vi "NI_PCIE_4353_32TC.vi"(11 "Queue Ref In":T1={"UI"=refnum, "Message"=refnum, "Data"=refnum, "Caller"=refnum, "Name"="000 Common", "Data Path"=path "", "Class Path"=path "", "SubPanel"=refnum, "Project Name"="", "MNT"="", "Title"="", "Data Source"=refnum, "Queue List"={}, "VI"=refnum, "UE"=refnum}) -> ()   [LabVIEW 2020]
doc: "PCIE_6509"
uses:
  Alin/QMH/000 Module Data Type.ctl
  Alin/QMH/Queue Message.ctl
  9999 SubVI/Global/Data Global/SDQ Data Type.ctl
  <vilib>/DAQmx/read.llb/DAQmx Read (Analog 1D DBL NChan 1Samp).vi
  <vilib>/DAQmx/create/channels.llb/DAQmx Create Channel (AI-Temperature-Thermocouple).vi
  <vilib>/DAQmx/miscellaneous.llb/DAQmx Fill In Error Info.vi
  <resource>/objmgr/daqmx.rc
panel:
  out "Type":map{string, string}(c390)
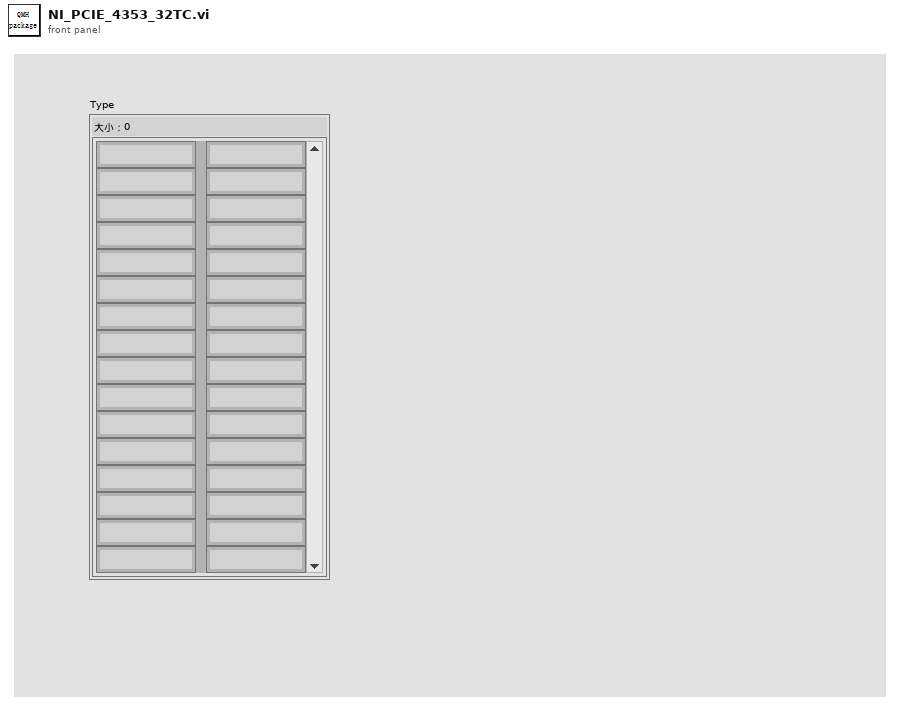
[diagram p1: front panel]
types:
  T1 = typedef "000 Module Data Type.ctl" = cluster{"UI":refnum<queue>, "Message":refnum<queue>, "Data":refnum<queue>, "Caller":refnum<queue>, "Name":string, "Data Path":path, "Class Path":path, "SubPanel":refnum<vi>, "Project Name":string, "MNT":string, "Title":string, "Data Source":refnum<queue>, "Queue List":map{string, refnum<queue>}, "VI":refnum<vi>, "UE":refnum<user-event>}
  T2 = typedef "SDQ Data Type.ctl" = cluster{"CAN Length":string, "CAN Name":string, "CAN ID":string, "CAN Type":string, "Test Item":string, "Byte Order":string, "Instruction":string, "Control Type":string, "Group":string, "Offset":dbl, "Coefficient":dbl, "Write Enable":bool, "Lable Type":string, "Key?":string, "Set Value":string, "Upper":dbl, "Lower":dbl, "Unit":string, "Formula":string, "Test Item Type":string, "Length":i32, "Address":string, "Name":string, "Identifier":string, "Data Type":string, "Enumerate?":string, "Enumerate List":string, "Data":string, "Source":string}
  T3 = cluster{"Queue":T1, "Delay":cluster{"Count Time(ms)":u32, "Delay Time(ms)":u32, "Next":string}, "Data":map{string, T2}, "PCIE_6509":cluster{"Port":string, "Task":refnum<k21>}, "IDS":string[], "Type":map{string, string}}
  T4 = typedef "005 Data Source Type.ctl" = cluster{"Device Name":string, "Device Model":string, "Device Driver":string, "IP Address":string, "Port":string, "Remark":string, "Enable":string, "Path":string}
  T5 = cluster{"Name":string, "Type":map{string, string}}
  T6 = typedef "eventvkey.ctl" = enum16{"ASCII", "Enter", "Return", "Shift", "Ctrl", "Alt", "Cmd", "Opt", "Caps", "NumLock", "Clear", "Break", "Up", "Down", "Left", "Right", "Insert", "Delete", "Home", "End", "PageUp", "PageDown", "Escape", "Help", "Pause", "ScrollLock", "F1", "F2", "F3", "F4", "F5", "F6", "F7", "F8", "F9", "F10", "F11", "F12", "F13", "F14", "F15", "F16", "F17", "F18", "F19", "F20", "F21", "F22", "F23", "F24", "Play", "VolumeUp", "VolumeDown", "Mute", "Two Byte Char"}
  T7 = cluster{"Shift":bool, "Ctrl":bool, "Alt":bool, "Cmd":bool, "Opt":bool}
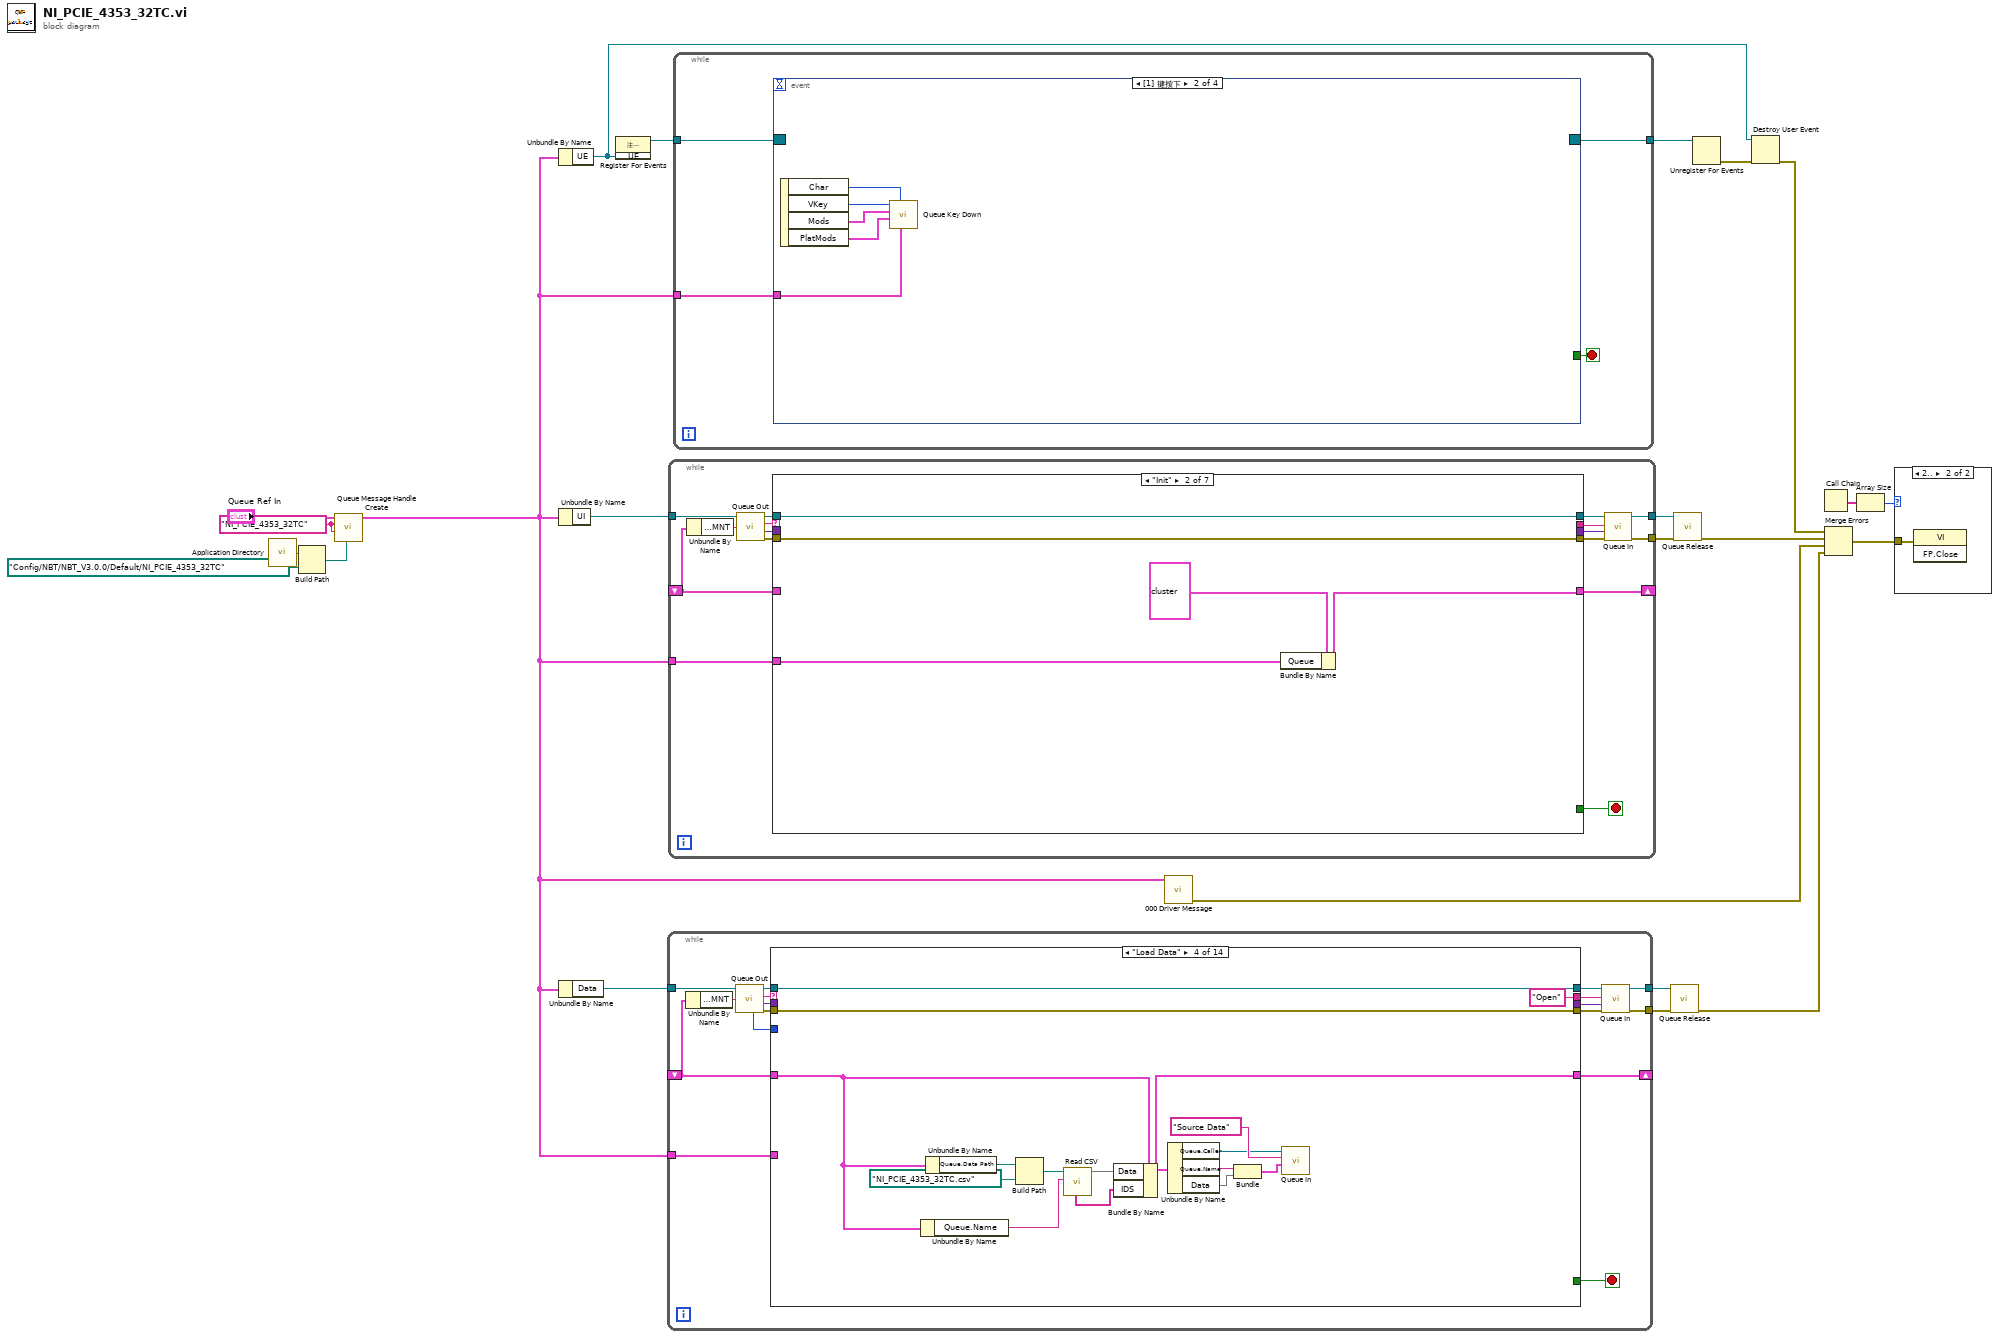
[diagram p0: block diagram]
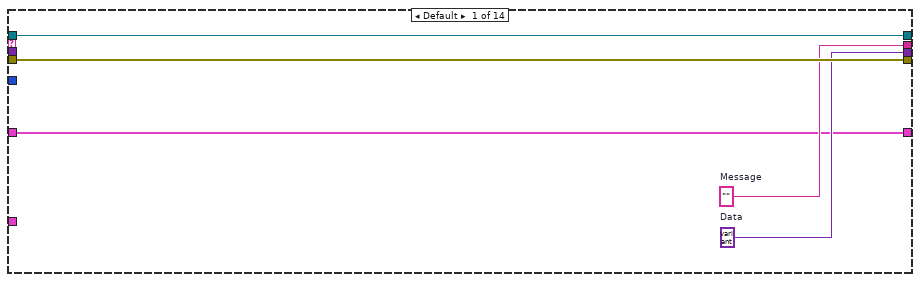
[diagram p2: hidden frame]
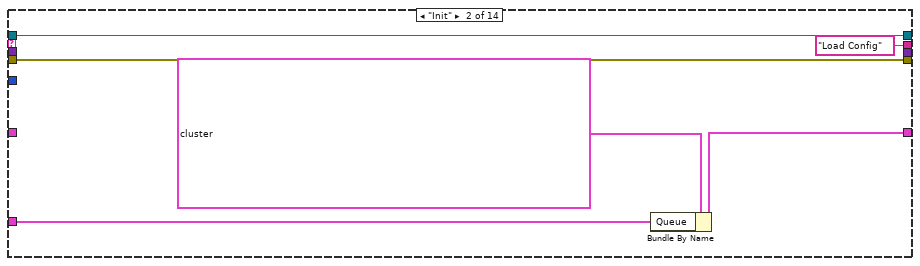
[diagram p3: hidden frame]
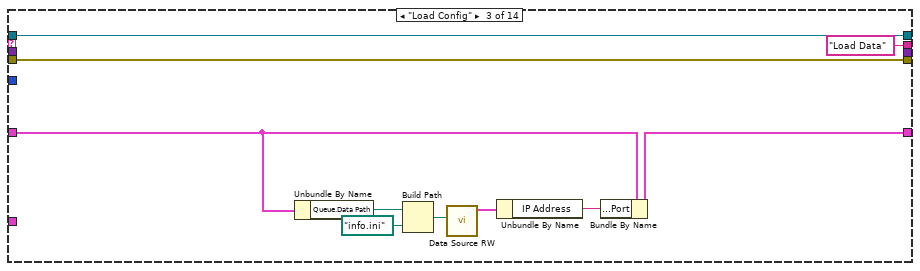
[diagram p4: hidden frame]
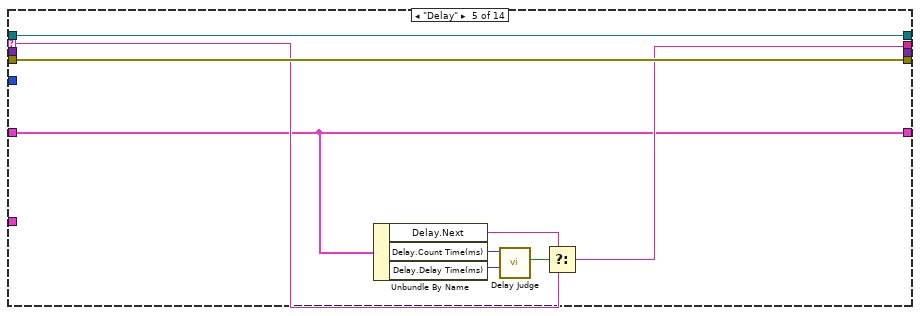
[diagram p5: hidden frame]
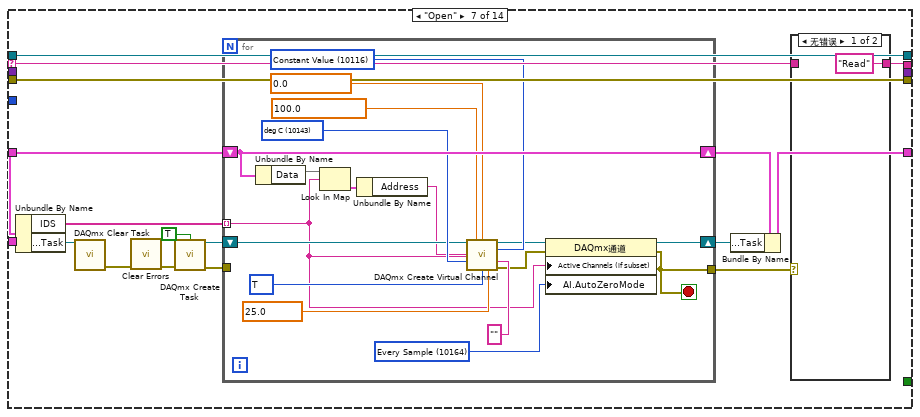
[diagram p7: hidden frame]
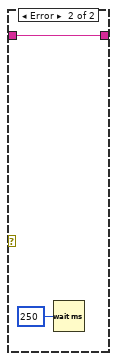
[diagram p8: hidden frame]
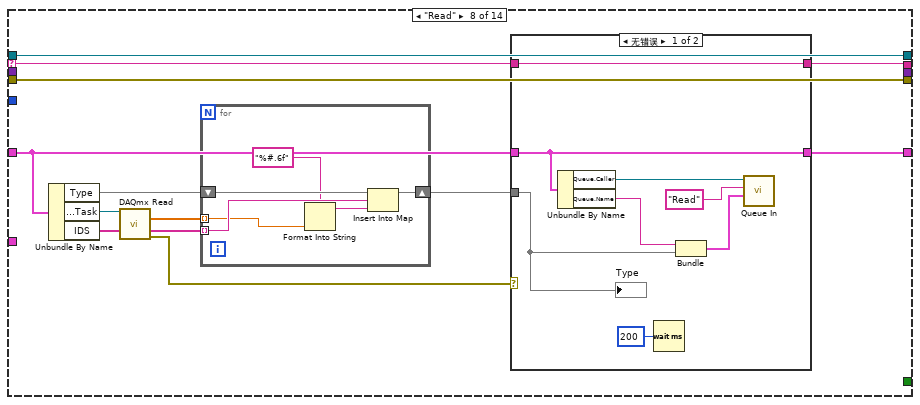
[diagram p9: hidden frame]
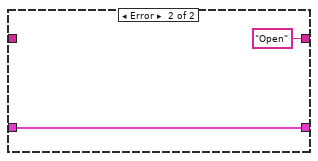
[diagram p10: hidden frame]
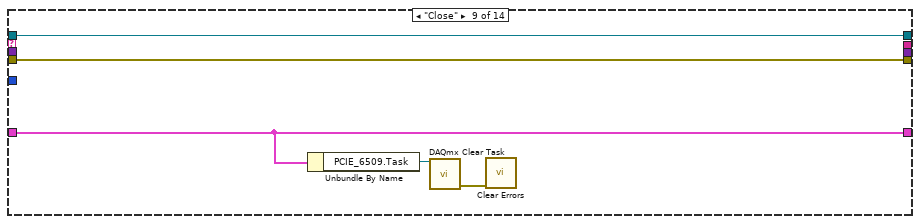
[diagram p11: hidden frame]
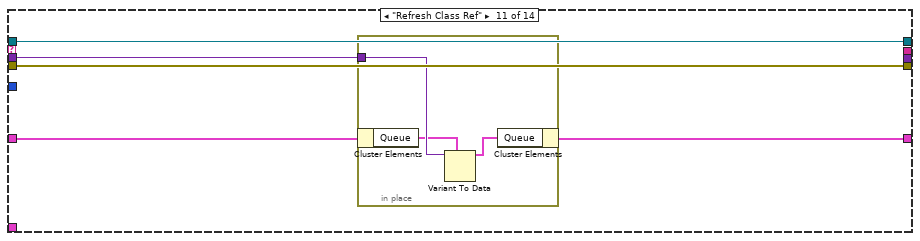
[diagram p13: hidden frame]
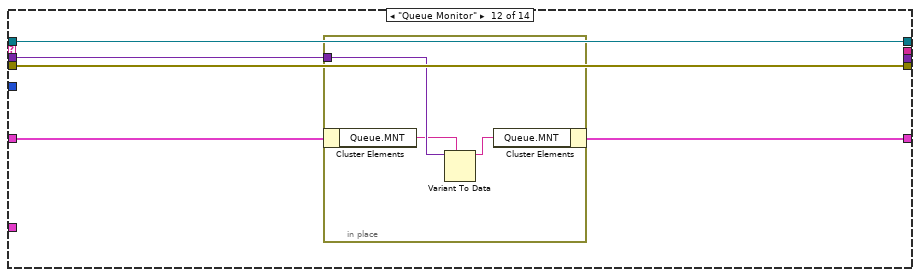
[diagram p14: hidden frame]
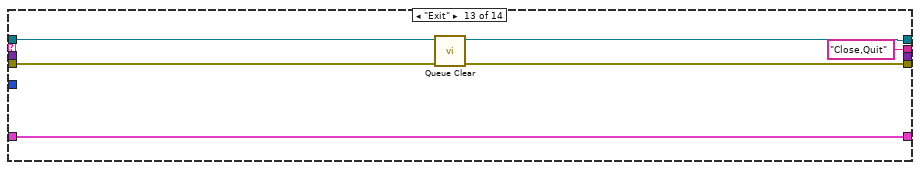
[diagram p15: hidden frame]
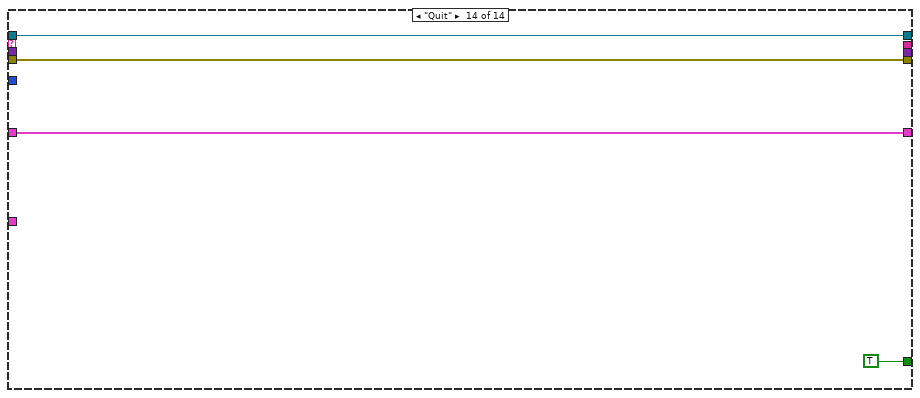
[diagram p16: hidden frame]
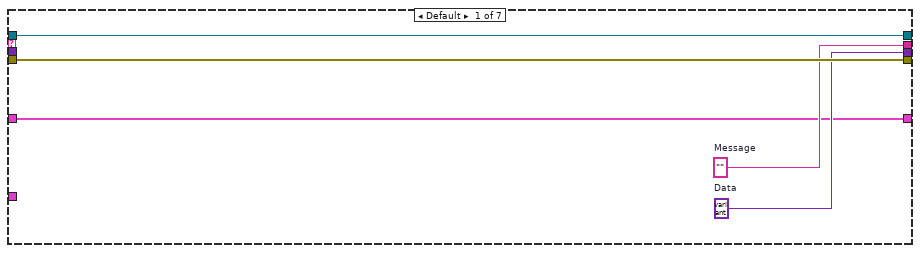
[diagram p18: hidden frame]
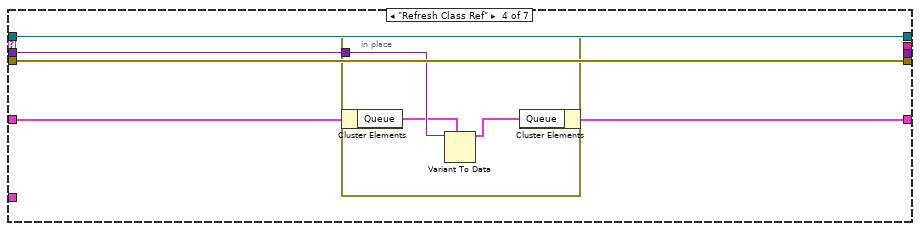
[diagram p20: hidden frame]
diagram:
  w1 = "NI_PCIE_4353_32TC" ("Title")
  n1 = call <vilib>:"Application Directory.vi"() -> ("Application Directory"=w4:path)
  n2 = Build Path(base path=w4, name or relative path=path "Config/NBT/NBT_V3.0.0/Default/NI_PCIE_4353_32TC" ("名称或相对路径")) -> (appended path=w2:path)
  n3 = call "Queue Message Handle Create.vi"("Data Path"=w2, "Name"=w1, "Title"=w1, "Queue Ref In"="Queue Ref In") -> ("Queue Ref Out"=w5:T1)  [unwired: 6 in, 1 out]
  n4 = Unbundle By Name(w5) -> ("UE"=w7:refnum<user-event>)
  n5 = Unbundle By Name(w5) -> ("UI"=w18:refnum<queue>)
  n6 = Unbundle By Name(w5) -> ("Data"=w10:refnum<queue>)
  n7 = register-events(w7) -> (reference out=w23:refnum<event-registration>)  [unwired: 2 in, 1 out]
  n8 = while {
    tunnel: w10 -> [w36]
    tunnel: [w33] -> w12
    tunnel: [w32] -> w11
    shift-right: [w28] -> _
    shift-left: _ -> [w25]
    tunnel: w5 -> [w24]
    stop <- w40 stop-if-true
    n9 = Unbundle By Name(w25) -> ("Queue.MNT"=w26:string)
    n10 = call "Queue Out.vi"("Monitor"=w26, "Queue In"=w36) -> ("error out"=w39:errorcluster, "Data"=w37:variant, "Message"=w38:string, "Queue Out"=w35:refnum<queue>, "Queue NUmber"=w27:i32)  [unwired: 5 in]
    n11 = case shown="\"Load Data\"" w38 {
      selector: w38 -> [_ _ _ _ w79 _ w95 w131 _ _ _ _ _ _]
      tunnel: w35 -> [w45 w51 w61 w77 w86 w89 w105 w138 w159 w162 w167 w175 w183 w187]
      tunnel: w39 -> [w44 w50 w60 w76 w85 w88 w104 w137 w158 w161 w166 w174 w181 w188]
      tunnel: [w45 w51 w61 w77 w86 w89 w105 w138 w159 w162 w167 w175 w182 w187] -> w34
      tunnel: [w44 w50 w60 w76 w85 w88 w104 w137 w158 w161 w166 w174 w180 w188] -> w31
      tunnel: [w43 "Load Config" ("Next") "Load Data" ("Next") "Open" ("Next") w80 _ w94 w130 _ _ _ _ "Close,Quit" _] -> w30
      tunnel: [_ _ _ _ _ _ _ _ _ _ _ _ _ TRUE] -> w40
      tunnel: [w42 _ _ _ _ _ _ _ _ _ _ _ _ _] -> w29
      tunnel: w37 -> [_ _ _ _ _ _ _ _ _ _ w163 w171 _ _]
      tunnel: [w41 w47 w53 w66 w78 w87 w102 w132 w157 w160 w164 w172 w179 w185] -> w28
      tunnel: w25 -> [w41 _ w58 w63 w78 w87 w92 w133 w157 w160 w165 w173 w179 w185]
      tunnel: w27 -> [_ _ _ _ _ _ _ _ _ _ _ _ _ _]
      tunnel: w24 -> [_ w46 _ _ _ _ _ _ _ _ _ _ _ _]
      frame Default {
        w42 = variant  # Data
        w43 = ""  # Message
      }
      frame "Init" {
        n12 = Bundle By Name(cluster=T3 {"Queue"={"UI"=refnum, "Message"=refnum, "Data"=refnum, "Caller"=refnum, "Name"="000 Common", "Data Path"=path "", "Class Path"=path "", "SubPanel"=refnum, "Project Name"="", "MNT"="", "Title"="", "Data Source"=refnum, "Queue List"={}, "VI"=refnum, "UE"=refnum}, "Delay"={"Count Time(ms)"=250, "Delay Time(ms)"=250, "Next"="Receive Data,Delay"}, "Data"={}, "PCIE_6509"={"Port"="", "Task"=""}, "IDS"=[], "Type"={}}, "Queue"=w46) -> (w47:T3)
      }
      frame "Load Config" {
        n13 = Unbundle By Name(w58) -> ("Queue.Data Path"=w57:path)
        n14 = Build Path(base path=w57, name or relative path=path "info.ini" ("名称或相对路径")) -> (appended path=w55:path)
        n15 = call "Data Source RW.vi"("Source Path"=w55) -> ("Data Type Out"=w54:T4)  [unwired: 7 in, 3 out]
        n16 = Unbundle By Name(w54) -> ("IP Address"=w52:string)
        n17 = Bundle By Name(cluster=w58, "PCIE_6509.Port"=w52) -> (w53:T3)
      }
      frame "Load Data" {
        n18 = Unbundle By Name(w63) -> ("Queue.Name"=w62:string)
        n19 = Unbundle By Name(w63) -> ("Queue.Data Path"=w75:path)
        n20 = Build Path(base path=w75, name or relative path=path "NI_PCIE_4353_32TC.csv" ("名称或相对路径")) -> (appended path=w73:path)
        n21 = call "Read CSV.vi"("Source"=w62, "Data Path"=w73) -> (3:"Identifiers Out"=w72:map{string, T2}, 6:"Identifiers Out"=w65:string[])  [unwired: 2 in, 6 out]
        n22 = Bundle By Name(cluster=w63, "Data"=w72, "IDS"=w65) -> (w66:T3)
        n23 = Unbundle By Name(w66) -> ("Queue.Caller"=w67:refnum<queue>, "Queue.Name"=w71:string, "Data"=w69:map{string, T2})
        n24 = Bundle("Name"=w71, "Data"=w69) -> (w70:cluster{"Name":string, "Data":map{string, T2}})  [unwired: 1 in]
        n25 = call "Queue In.vi"("Data"=w70, "Message"="Source Data", "Queue In"=w67) -> ()  [unwired: 7 in, 2 out]
      }
      frame "Delay" {
        n26 = Unbundle By Name(w78) -> ("Delay.Next"=w84:string, "Delay.Count Time(ms)"=w81:u32, "Delay.Delay Time(ms)"=w82:u32)
        n27 = call "Delay Judge.vi"("Delay Time(ms)"=w82, "Count Time(ms)"=w81) -> ("Time Out?"=w83:bool)  [unwired: 5 in, 4 out]
        n28 = Select(t=w84, s=w83, f=w79) -> (s? t:f=w80:string)
      }
      frame "===Driver====" {
      }
      frame "Open" {
        n29 = Unbundle By Name(w92) -> ("IDS"=w93:string[], "PCIE_6509.Task"=w101:refnum<k21>)
        n30 = call <vilib>:"DAQmx Clear Task.vi"("task in"=w101) -> ("error out"=w100:errorcluster)  [unwired: 14 in]
        n31 = call <vilib>:"Clear Errors.vi"("error in (no error)"=w100) -> ("error out"=w99:errorcluster)  [unwired: 5 in, 1 out]
        n32 = call <vilib>:"DAQmx Create Task.vi"("auto cleanup"=TRUE, "error in"=w99) -> ("task out"=w98:refnum<k21>, "error out"=w90:errorcluster)  [unwired: 12 in]
        n33 = for {
          shift-right: [w113] -> w97
          shift-left: w98 -> [w116]
          tunnel: [w111] -> w96
          tunnel: w93 -> [w110] mode=indexing
          shift-right: [w126] -> w91
          shift-left: w92 -> [w126]
          tunnel: w90 -> [_]
          stop <- w111 stop-if-true
          w109 = 10164 items=["None"=10230, "Once"=10244, "Every Sample"=10164] ("AutoZeroMode")
          w120 = 10143 items=["deg C"=10143, "deg F"=10144, "Kelvins"=10325, "deg R"=10145, "From Custom Scale"=10065] ("units")
          w118 = 10086 items=["J"=10072, "K"=10073, "N"=10077, "R"=10082, "S"=10085, "T"=10086, "B"=10047, "E"=10055] ("thermocouple type")
          w121 = u32 10116 items=["Internal"=10200, "Constant Value"=10116, "Channel"=10113] ("cjc source")
          n34 = Unbundle By Name(w126) -> ("Data"=w125:map{string, T2})
          n35 = Look In Map(map=w125, key=w110) -> (value=w124:T2)  [unwired: 1 in, 1 out]
          n36 = Unbundle By Name(w124) -> ("Address"=w115:string)
          n37 = call-poly <vilib>:"DAQmx Create Virtual Channel.vi"("task in"=w116, "maximum value"=100.0, "minimum value"=0.0, "physical channels"=w115, "cjc source"=w121, "name to assign"=w110, "units"=w120, "cjc channel"="", "thermocouple type"=w118, "cjc value"=25.0) -> ("task out"=w114:refnum<k21>, "error out"=w112:errorcluster)  [unwired: 4 in]
          n38 = property class="DAQmx通道"(reference=w114, error in=w112, "Active Channels (if subset)"=w110, "AI.AutoZeroMode"=w109) -> (reference out=w113:refnum<k21>, error out=w111:errorcluster)
        }
        n39 = Bundle By Name(cluster=w91, "PCIE_6509.Task"=w97) -> (w102:T3)
        n40 = case shown="无错误" w96 {
          tunnel: w95 -> [_ w108]
          tunnel: ["Read" w108] -> w94
          frame No Error {
          }
          frame Error {
            n41 = Wait (ms)(milliseconds to wait=u32 250 ("等待时间（毫秒）")) -> ()  [unwired: 1 out]
          }
        }
      }
      frame "Read" {
        n42 = Unbundle By Name(w133) -> ("Type"=w135:map{string, string}, "PCIE_6509.Task"=w129:refnum<k21>, "IDS"=w136:string[])
        n43 = call-poly <vilib>:"DAQmx Read.vi"("task/channels in"=w129) -> ("data"=w127:dbl[], "error out"=w128:errorcluster)  [unwired: 12 in, 1 out]
        n44 = for {
          tunnel: w136 -> [w153] mode=indexing
          shift-right: [w152] -> w134
          shift-left: w135 -> [w154]
          tunnel: w127 -> [w150] mode=indexing
          n45 = Format Into String(format string="%#.6f" ("格式字符串"), w150) -> (resulting string=w149:string)  [unwired: 2 in, 1 out]
          n46 = Insert Into Map(map in=w154, key=w153, value=w149) -> (map out=w152:map{string, string})  [unwired: 2 out]
        }
        n47 = case shown="无错误" w128 {
          tunnel: w134 -> [w139 _]
          tunnel: w133 -> [w146 w148]
          tunnel: [w146 w148] -> w132
          tunnel: w131 -> [w141 _]
          tunnel: [w141 "Open"] -> w130
          frame No Error {
            n48 = Unbundle By Name(w146) -> ("Queue.Caller"=w145:refnum<queue>, "Queue.Name"=w143:string)
            n49 = Wait (ms)(milliseconds to wait=u32 200 ("等待时间（毫秒）")) -> ()  [unwired: 1 out]
            n50 = Bundle("Name"=w143, "Type"=w139) -> (w142:T5)  [unwired: 1 in]
            n51 = call "Queue In.vi"("Data"=w142, "Message"="Read", "Queue In"=w145) -> ()  [unwired: 7 in, 2 out]
            "Type" <- w139
          }
          frame Error {
          }
        }
      }
      frame "Close" {
        n52 = Unbundle By Name(w157) -> ("PCIE_6509.Task"=w156:refnum<k21>)
        n53 = call <vilib>:"DAQmx Clear Task.vi"("task in"=w156) -> ("error out"=w155:errorcluster)  [unwired: 14 in]
        n54 = call <vilib>:"Clear Errors.vi"("error in (no error)"=w155) -> ()  [unwired: 5 in, 2 out]
      }
      frame "====System====" {
      }
      frame "Refresh Class Ref" {
        n55 = in-place {
          in-place-border: w163 -> [w170]
          n56 = in-place-cluster #1(w165) -> ("Queue"=w169:T1)
          n57 = Variant To Data(type=w169, Variant=w170) -> (data=w168:T1)  [unwired: 1 in, 1 out]
          n58 = in-place-cluster #1("Queue"=w168) -> (w164:T3)
        }
      }
      frame "Queue Monitor" {
        n59 = in-place {
          in-place-border: w171 -> [w178]
          n60 = in-place-cluster #2(w173) -> ("Queue.MNT"=w177:string)
          n61 = Variant To Data(type=w177, Variant=w178) -> (data=w176:string)  [unwired: 1 in, 1 out]
          n62 = in-place-cluster #2("Queue.MNT"=w176) -> (w172:T3)
        }
      }
      frame "Exit" {
        n63 = call "Queue Clear.vi"("error in (no error)"=w181, "Queue In"=w183) -> ("error out"=w180:errorcluster, "Queue Out"=w182:refnum<queue>)  [unwired: 8 in]
      }
      frame "Quit" {
      }
    }
    n64 = call "Queue In.vi"("error in (no error)"=w31, "Data"=w29, "Message"=w30, "Queue In"=w34) -> ("error out"=w32:errorcluster, "Queue Out"=w33:refnum<queue>)  [unwired: 6 in]
  }
  n65 = while {
    tunnel: w18 -> [w200]
    tunnel: [w197] -> w20
    tunnel: [w196] -> w19
    shift-right: [w192] -> _
    shift-left: _ -> [w191]
    tunnel: w5 -> [w189]
    stop <- w204 stop-if-true
    n66 = Unbundle By Name(w191) -> ("Queue.MNT"=w190:string)
    n67 = call "Queue Out.vi"("Monitor"=w190, "Queue In"=w200) -> ("error out"=w203:errorcluster, "Data"=w201:variant, "Message"=w202:string, "Queue Out"=w199:refnum<queue>)  [unwired: 5 in, 1 out]
    n68 = case shown="\"Init\"" w202 {
      selector: w202 -> [_ _ _ _ _ w236 _]
      tunnel: w199 -> [w209 w214 w217 w222 w230 w243 w249]
      tunnel: w203 -> [w208 w213 w216 w221 w229 w241 w250]
      tunnel: [w209 w214 w217 w222 w230 w242 w249] -> w198
      tunnel: [w208 w213 w216 w221 w229 w240 w250] -> w195
      tunnel: [w207 _ _ _ _ "Quit" _] -> w194
      tunnel: [_ _ _ _ _ _ TRUE] -> w204
      tunnel: [w206 _ _ _ _ _ _] -> w193
      tunnel: w201 -> [_ _ _ w218 w226 _ _]
      tunnel: [w205 w211 w215 w219 w227 w235 w247] -> w192
      tunnel: w191 -> [w205 _ w215 w220 w228 w235 w247]
      tunnel: w189 -> [_ w210 _ _ _ _ _]
      frame Default {
        w206 = variant  # Data
        w207 = ""  # Message
      }
      frame "Init" {
        n69 = Bundle By Name(cluster=cluster{"Queue":T1} {"Queue"={"UI"=refnum, "Message"=refnum, "Data"=refnum, "Caller"=refnum, "Name"="000 Common", "Data Path"=path "", "Class Path"=path "", "SubPanel"=refnum, "Project Name"="", "MNT"="", "Title"="", "Data Source"=refnum, "Queue List"={}, "VI"=refnum, "UE"=refnum}}, "Queue"=w210) -> (w211:cluster{"Queue":T1})
      }
      frame "====System====" {
      }
      frame "Refresh Class Ref" {
        n70 = in-place {
          in-place-border: w218 -> [w225]
          n71 = in-place-cluster #3(w220) -> ("Queue"=w224:T1)
          n72 = Variant To Data(type=w224, Variant=w225) -> (data=w223:T1)  [unwired: 1 in, 1 out]
          n73 = in-place-cluster #3("Queue"=w223) -> (w219:cluster{"Queue":T1})
        }
      }
      frame "Queue Monitor" {
        n74 = in-place {
          in-place-border: w226 -> [w233]
          n75 = in-place-cluster #4(w228) -> ("Queue.MNT"=w232:string)
          n76 = Variant To Data(type=w232, Variant=w233) -> (data=w231:string)  [unwired: 1 in, 1 out]
          n77 = in-place-cluster #4("Queue.MNT"=w231) -> (w227:cluster{"Queue":T1})
        }
      }
      frame "Exit" {
        n78 = Unbundle By Name(w235) -> ("Queue.Message"=w239:refnum<queue>, "Queue.Data"=w238:refnum<queue>, "Queue.UE"=w234:refnum<user-event>)
        n79 = Build Array(w239, w238) -> (w237:refnum<queue>[])
        n80 = Generate User Event(user event=w234, event data cluster=w236) -> ()  [unwired: 2 in, 2 out]
        n81 = for {
          tunnel: w237 -> [w246] mode=indexing
          tunnel: w236 -> [w245]
          n82 = call "Queue In.vi"("Message"=w245, "Queue In"=w246) -> ()  [unwired: 8 in, 2 out]
        }
        n83 = call "Queue Clear.vi"("error in (no error)"=w241, "Queue In"=w243) -> ("error out"=w240:errorcluster, "Queue Out"=w242:refnum<queue>)  [unwired: 8 in]
      }
      frame "Quit" {
      }
    }
    n84 = call "Queue In.vi"("error in (no error)"=w195, "Data"=w193, "Message"=w194, "Queue In"=w198) -> ("error out"=w196:errorcluster, "Queue Out"=w197:refnum<queue>)  [unwired: 6 in]
  }
  n85 = while {
    tunnel: w23 -> [w254]
    tunnel: [w252] -> w22
    tunnel: w5 -> [w251]
    stop <- w253 stop-if-true
    n86 = event shown="[1] 键按下" {
      selector: w254 -> [_ _ _ _]
      dyn-events: [_ _ _ _] -> w252
      timeout: _ -> [_ _ _ _]
      tunnel: [_ _ w260 _] -> w253
      tunnel: w251 -> [_ w255 _ w265]
      event Timeout {
        n87 = event-data() -> ()  [unwired: 1 in, 1 out]
      }
      event Key Down {
        n88 = event-data() -> ("Char"=w259:i16, "VKey"=w258:T6, "Mods"=w257:cluster{"Num Pad":bool, "Menu Key":bool}, "PlatMods"=w256:T7)  [unwired: 1 in]
        n89 = call "Queue Key Down.vi"("Queue Ref Out"=w255, "C"=w259, "Platform Key"=w256, "Group Key"=w257, "V Key"=w258) -> ()  [unwired: 6 in, 1 out]
      }
      event User Event {
        n90 = event-data() -> ("Message"=w262:string)  [unwired: 1 in]
        n91 = Equal?(x=w262, y="Exit") -> (x = y?=w260:bool)
      }
      event Panel Close? {
        n92 = event-data() -> ()  [unwired: 1 in, 1 out]
        n93 = Call Chain() -> (call chain=w267:string[])
        n94 = Array Size(array=w267) -> (size(s)=w266:i32)
        n95 = case shown="2, 默认" w266 {
          tunnel: w265 -> [w271 w274]
          tunnel: [w270 w273] -> w264
          tunnel: ["Panel Hidden" ("Message") "Exit Prepare" ("Message")] -> w263
          frame 2, Default {
            n96 = Unbundle By Name(w271) -> ("Message"=w270:refnum<queue>)
          }
          frame 1 {
            n97 = Unbundle By Name(w274) -> ("Message"=w273:refnum<queue>)
          }
        }
        n98 = call "Queue In.vi"("Message"=w263, "Queue In"=w264) -> ()  [unwired: 8 in, 2 out]
        n99 = event-data("Discard?"=TRUE ("放弃？")) -> ()  [unwired: 1 in, 1 out]
      }
    }
  }
  n100 = call "000 Driver Message.vi"("Queue In"=w5) -> ("error out"=w8:errorcluster)  [unwired: 8 in, 2 out]
  n101 = call "Queue Release.vi"("error in (no error)"=w11, "Queue In"=w12) -> ("error out"=w9:errorcluster)  [unwired: 9 in]
  n102 = call "Queue Release.vi"("error in (no error)"=w19, "Queue In"=w20) -> ("error out"=w16:errorcluster)  [unwired: 9 in]
  n103 = Unregister For Events(event registration refnum=w22) -> (error out=w21:errorcluster)  [unwired: 1 in]
  n104 = Destroy User Event(user event=w7, error in=w21) -> (error out=w17:errorcluster)
  n105 = Call Chain() -> (call chain=w14:string[])
  n106 = Merge Errors(w17, w16, w8, w9) -> (w15:errorcluster)
  n107 = Array Size(array=w14) -> (size(s)=w13:i32)
  n108 = case shown="2.." w13 {
    tunnel: w15 -> [_ w275]
    frame 0, Default {
    }
    frame 2.. {
      n109 = invoke class="VI" method="FP.Close"(error in=w275) -> ()  [unwired: 2 in, 3 out]
    }
  }
